vi "Find Best Settings.vi"() -> ()   [LabVIEW 2020]
uses:
  2aca6401-861b-43a8-89dd-559ac588650a.vi
  0d72e569-569c-4e7b-9da6-a5ac3a5322a1.vi
  <vilib>/Array/Sort 2D Array - Pop Stack.vi
  <vilib>/Array/Sort 2D Array - Push Stack.vi
  2aca6401-861b-43a8-89dd-559ac588650a.vi/269d4b3b-47f5-49e3-8884-44851e4dd9d5.vi
  2aca6401-861b-43a8-89dd-559ac588650a.vi/6d99389c-673d-4efb-bf33-19b32bcf4cf8.vi
panel:
  out "Sorted Settings":string[][](array[string])
  out "Best Settings":string[](array[string])
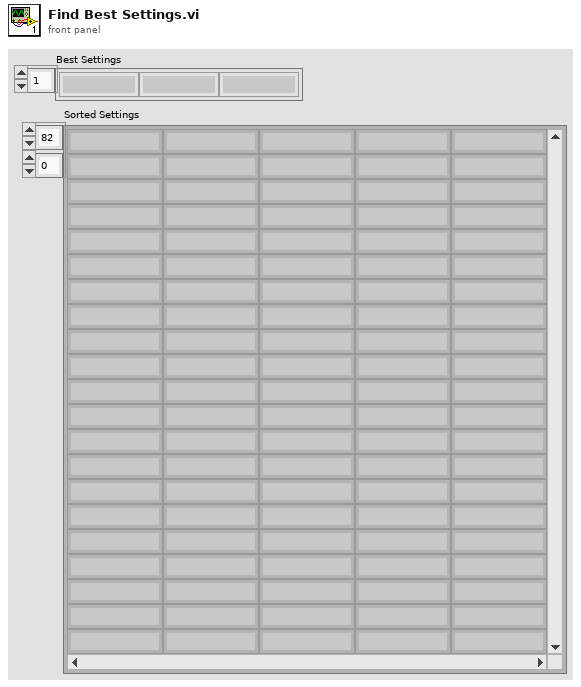
[diagram p1: front panel]
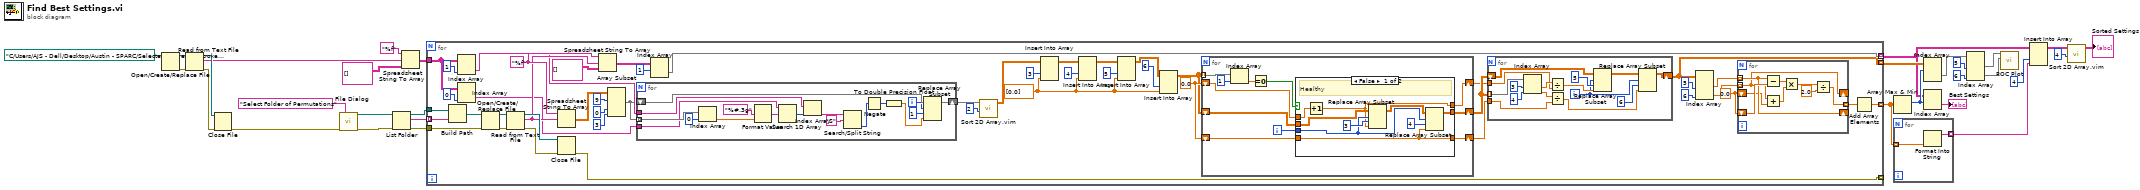
[diagram p0: block diagram]
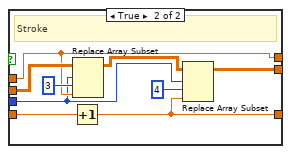
[diagram p2: hidden frame]
diagram:
  n1 = Open/Create/Replace File(file path (use dialog)=path "C:/Users/AJS - Dell/Desktop/Austin - SPARC/Selected Subjects - Stroke Analysis/Subject Groups.txt") -> (refnum out=w22:refnum<file>, error out=w21:errorcluster)  [unwired: 5 in, 1 out]
  n2 = Read from Text File(file (use dialog)=w22, error in=w21) -> (refnum out=w23:refnum<file>, text=w19:string, error out=w24:errorcluster)  [unwired: 2 in, 1 out]
  n3 = Close File(refnum=w23, error in=w24) -> (error out=w16:errorcluster)  [unwired: 1 out]
  n4 = call "File Dialog"("prompt"="Select Folder of Permutations", "error in"=w16) -> ("selected path"=w31:path, "error out"=w30:errorcluster)  [unwired: 10 in, 2 out]
  n5 = List Folder(path=w31, error in=w30) -> (path out=w27:path, filenames=w29:string[], error out=w28:errorcluster)  [unwired: 2 in, 1 out]
  n6 = Spreadsheet String To Array(format string="%f", spreadsheet string=w19, array type (2D Dbl)=string[][] []) -> (array=w17:string[][])  [unwired: 1 in]
  n7 = for {
    tunnel: w29 -> [w79] mode=indexing
    tunnel: w28 -> [w80]
    tunnel: w27 -> [w78]
    tunnel: [w69] -> w4 mode=indexing
    tunnel: [w68] -> _ mode=indexing
    tunnel: [w39] -> w8 mode=indexing
    tunnel: w17 -> [w58]
    tunnel: [w32] -> w7 mode=indexing
    w34 = 0.0
    w46 = dbl[] [0.0] ("new element/subarray")
    w53 = 0.0
    w67 = "%f" ("format string")
    n8 = Build Path(base path=w78, name or relative path=w79) -> (appended path=w75:path)
    n9 = Index Array(array=w58, index (col)=1 ("disabled index (col)")) -> (element=w56:string[])  [unwired: 1 in]
    n10 = Index Array(array=w58, index (col)=0 ("disabled index (col)")) -> (element=w59:string[])  [unwired: 1 in]
    n11 = Open/Create/Replace File(file path (use dialog)=w75, error in=w80) -> (refnum out=w73:refnum<file>, error out=w76:errorcluster)  [unwired: 4 in, 1 out]
    n12 = Read from Text File(file (use dialog)=w73, error in=w76) -> (refnum out=w77:refnum<file>, text=w66:string, error out=w74:errorcluster)  [unwired: 2 in, 1 out]
    n13 = Spreadsheet String To Array(format string=w67, spreadsheet string=w66) -> (array=w65:dbl[][])  [unwired: 2 in]
    n14 = Close File(refnum=w77, error in=w74) -> (error out=w68:errorcluster)  [unwired: 1 out]
    n15 = Spreadsheet String To Array(format string=w67, spreadsheet string=w66, array type (2D Dbl)=string[][] []) -> (array=w70:string[][])  [unwired: 1 in]
    n16 = Array Subset(array=w65, index (row)=9 ("index"), index (col)=0 ("index"), length (col)=3 ("length")) -> (w55:dbl[][])  [unwired: 1 in]
    n17 = for {
      tunnel: w59 -> [w149]
      tunnel: w55 -> [w150] mode=indexing
      tunnel: w56 -> [w145]
      shift-right: [w140] -> w54
      shift-left: w55 -> [w143]
      i -> [w142]
      n18 = Index Array(array=w150, index=0) -> (element=w148:dbl)
      n19 = Format Value(format string="%#.3g", value (0)=w148) -> (output string=w147:string)  [unwired: 1 in]
      n20 = Search 1D Array(1D array=w149, element=w147) -> (index of element=w144:i32)  [unwired: 1 in]
      n21 = Index Array(array=w145, index=w144) -> (element=w139:string)
      n22 = Search/Split String(string=w139, search string/char (-)="S") -> (offset of match=w134:i32)  [unwired: 1 in, 2 out]
      n23 = Negate(x=w134) -> (-x=w136:i32)
      n24 = To Double Precision Float(number=w136) -> (double precision float=w137:dbl)
      n25 = Replace Array Subset(array=w143, new element=w137, index (row)=w142, index (col)=1 ("disabled index (col)")) -> (w140:dbl[][])
    }
    n26 = Index Array(array=w70, index (row)=1) -> (element=w69:string[])  [unwired: 1 in]
    n27 = call "Sort 2D Array.vim"("index"=2, "2D array"=w54) -> ("sorted 2D array"=w52:dbl[][])  [unwired: 8 in, 1 out]
    n28 = Insert Into Array(array=w52, index (col)=3 ("disabled index (col)"), new element=w46) -> (w50:dbl[][])  [unwired: 1 in]
    n29 = Insert Into Array(array=w50, index (col)=4 ("disabled index (col)"), new element=w46) -> (w43:dbl[][])  [unwired: 1 in]
    n30 = Insert Into Array(array=w43, index (col)=5 ("disabled index (col)"), new element=w46) -> (w44:dbl[][])  [unwired: 1 in]
    n31 = Insert Into Array(array=w44, index (col)=6 ("disabled index (col)"), new element=w46) -> (w45:dbl[][])  [unwired: 1 in]
    n32 = for {
      tunnel: w45 -> [w115] mode=indexing
      shift-right: [w110] -> w41
      shift-left: w53 -> [w111]
      shift-right: [w108] -> w40
      shift-left: w53 -> [w109]
      shift-right: [w105] -> w42
      shift-left: w45 -> [w107]
      i -> [w106]
      n33 = Index Array(array=w115, index=1) -> (element=w113:dbl)
      n34 = Equal To 0?(x=w113) -> (x = 0?=w112:bool)
      n35 = case shown="False" w112 {
        tunnel: w111 -> [w124 w130]
        tunnel: [w116 w130] -> w110
        tunnel: w109 -> [w117 w133]
        tunnel: [w117 w126] -> w108
        tunnel: w107 -> [w123 w132]
        tunnel: w106 -> [w119 w128]
        tunnel: [w120 w125] -> w105
        frame False {
          # "Healthy"
          n36 = Increment(x=w124) -> (x+1=w116:dbl)
          n37 = Replace Array Subset(array=w123, new element=w116, index (row)=w119, index (col)=3 ("disabled index (col)")) -> (w121:dbl[][])
          n38 = Replace Array Subset(array=w121, new element=w117, index (row)=w119, index (col)=4 ("disabled index (col)")) -> (w120:dbl[][])
        }
        frame True {
          # "Stroke"
          n39 = Increment(x=w133) -> (x+1=w126:dbl)
          n40 = Replace Array Subset(array=w132, new element=w130, index (row)=w128, index (col)=3 ("disabled index (col)")) -> (w129:dbl[][])
          n41 = Replace Array Subset(array=w129, new element=w126, index (row)=w128, index (col)=4 ("disabled index (col)")) -> (w125:dbl[][])
        }
      }
    }
    n42 = for {
      shift-right: [w93] -> w39
      shift-left: w42 -> [w97]
      tunnel: w42 -> [w104] mode=indexing
      tunnel: w41 -> [w101]
      tunnel: w40 -> [w99]
      i -> [w91]
      n43 = Index Array(array=w104, index #1=3 ("index"), index #2=4 ("index")) -> (element #1=w102:dbl, element #2=w98:dbl)
      n44 = Divide(x=w102, y=w101) -> (x/y=w96:dbl)
      n45 = Divide(x=w98, y=w99) -> (x/y=w92:dbl)
      n46 = Replace Array Subset(array=w97, new element=w96, index (row)=w91, index (col)=5 ("disabled index (col)")) -> (w94:dbl[][])
      n47 = Replace Array Subset(array=w94, new element=w92, index (row)=w91, index (col)=6 ("disabled index (col)")) -> (w93:dbl[][])
    }
    n48 = Index Array(array=w39, index (col) #1=5 ("disabled index (col)"), index (col) #2=6 ("disabled index (col)")) -> (element #1=w36:dbl[], element #2=w35:dbl[])  [unwired: 2 in]
    n49 = for {
      tunnel: w36 -> [w84] mode=indexing
      tunnel: w35 -> [w83] mode=indexing
      tunnel: [w88] -> w33 mode=indexing
      shift-right: [w84] -> _
      shift-left: w34 -> [w85]
      shift-right: [w83] -> _
      shift-left: w34 -> [w82]
      n50 = Subtract(x=w84, y=w85) -> (x-y=w86:dbl)
      n51 = Add(x=w83, y=w82) -> (x+y=w81:dbl)
      n52 = Multiply(x=w86, y=w81) -> (x*y=w89:dbl)
      n53 = Divide(x=w89, y=2.0) -> (x/y=w88:dbl)
    }
    n54 = Add Array Elements(numeric array=w33) -> (sum=w32:dbl)
  }
  n55 = Array Max & Min(array=w7) -> (max index (indices)=w10:i32)  [unwired: 3 out]
  n56 = for {
    tunnel: w7 -> [w152] mode=indexing
    tunnel: [w151] -> w1 mode=indexing
    n57 = Format Into String(w152) -> (resulting string=w151:string)  [unwired: 3 in, 1 out]
  }
  n58 = Index Array(array=w8, index (dim 0)=w10) -> (element=w15:dbl[][])  [unwired: 2 in]
  n59 = Index Array(array=w4, index (row)=w10) -> (element=→"Best Settings":string[])  [unwired: 1 in]
  n60 = Index Array(array=w15, index (col) #1=5 ("disabled index (col)"), index (col) #2=6 ("index (col)")) -> (element #1=w12:dbl[], element #2=w11:dbl[])  [unwired: 2 in]
  n61 = call "ROC Plot.vi"("Sens."=w11, "1-Spec."=w12) -> ()  [unwired: 10 in]
  n62 = Insert Into Array(array=w4, index (col)=4 ("disabled index (col)"), new element=w1) -> (w3:string[][])  [unwired: 1 in]
  n63 = call "Sort 2D Array.vim"("index"=4, "2D array"=w3) -> ("sorted 2D array"=→"Sorted Settings":string[][])  [unwired: 8 in, 1 out]
